vi "Disconnect.vi"(10 "error in (no error)":errorcluster, 11 "ICommHandler in":refnum<class "ICommHandler.lvclass">) -> (2 "error out":errorcluster, 3 "ICommHandler out":refnum<class "ICommHandler.lvclass">)   [LabVIEW 2020, in "wamplv.lvlib" / "ICommHandler.lvclass"]
uses:
  <vilib>/samangh/wamplv/Comm Handlers/ICommHandler/ICommHandler.lvclass
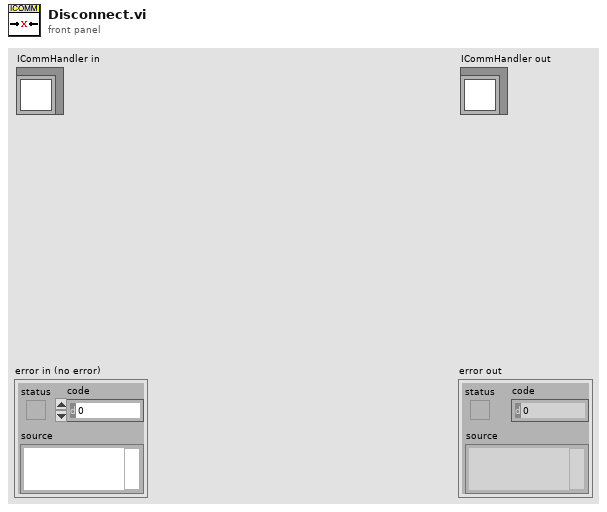
[diagram p1: front panel]
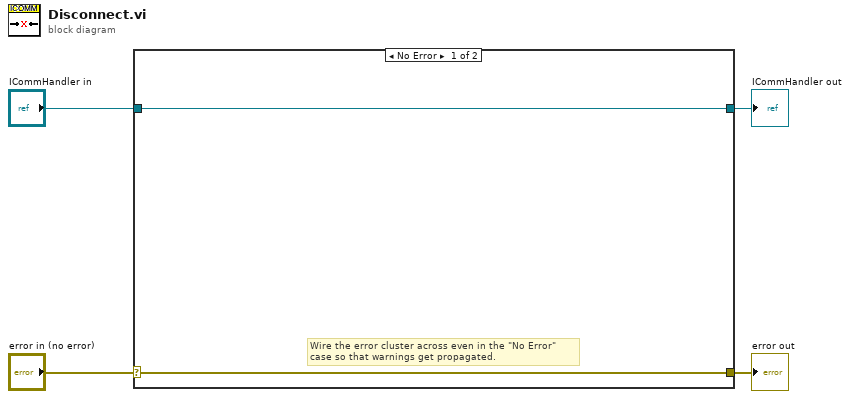
[diagram p0: block diagram]
diagram:
  n1 = case shown="No Error" "error in (no error)" {
    selector: "error in (no error)" -> [w5 w8]
    tunnel: [w5 w8] -> w3
    tunnel: [w6 w7] -> w1
    tunnel: "ICommHandler in" -> [w6 w7]
    frame No Error {
      # "Wire the error cluster across even in the \"No Error\"\ncase so that warnings get propagated."
    }
    frame Error {
    }
  }
  "error out" <- w3
  "ICommHandler out" <- w1
